vi "open_stream.vi"(6 "configuration":u64, 8 "buffer_size":u64, 9 "port":u16, 10 "host":string, 11 "path in":path=path "hl2ss_ulm.dll") -> (0 "buffer_size":u64, 1 "port":u16, 2 "host":string, 3 "path out":path, 4 "configuration":u64, 5 "handle":u64)   [LabVIEW 2023]
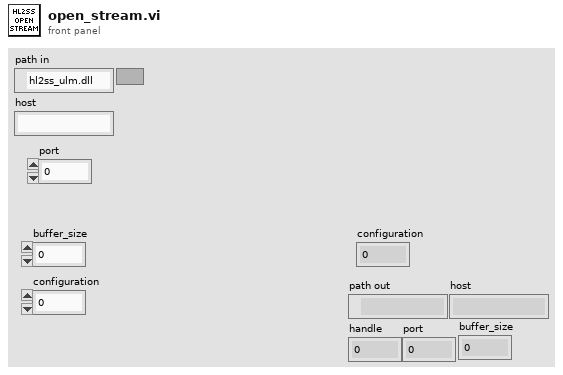
[diagram p1: front panel]
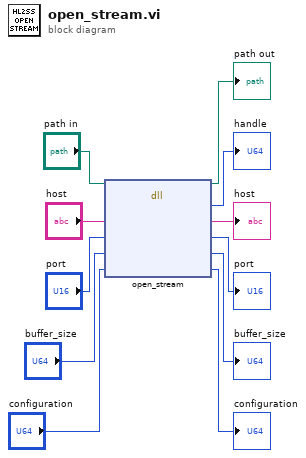
[diagram p0: block diagram]
diagram:
  n1 = dll-call lib="C:/Users/jcds/Documents/GitHub/hl2ss/extensions/client_labview/hl2ss_ulm.dll" fn="open_stream"(path in="path in", "host"="host", "port"="port", "buffer_size"="buffer_size", "configuration"="configuration") -> (path out=→"path out":path, "return type"=→"handle":u64, "host"=→"host":string, "port"=→"port":u16, "buffer_size"=→"buffer_size":u64, "configuration"=→"configuration":u64)  [unwired: 2 in, 1 out]
